vi "ShortCutForControlAndInd.vi"() -> ()   [LabVIEW 2019]
panel:
  out "x+y":dbl
  in  "x":dbl
  in  "y":dbl
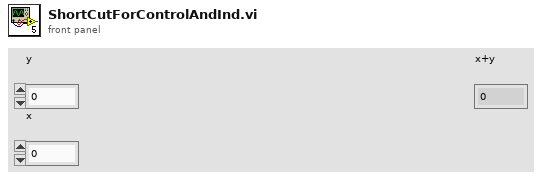
[diagram p1: front panel]
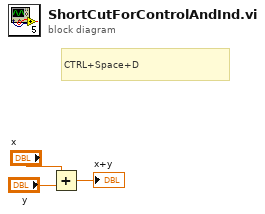
[diagram p0: block diagram]
diagram:
  # "CTRL+Space+D"
  n1 = Add(x="x", y="y") -> (x+y=→"x+y":dbl)
